vi "Disconnect PV.vi"(8 "error in (no error)":errorcluster, 10 "PV URL":string, 11 "CS++DIMCommandMonitor in":refnum<class "CS++DIMCommandMonitor.lvclass">) -> (0 "error out":errorcluster, 3 "CS++DIMCommandMonitor out":refnum<class "CS++DIMCommandMonitor.lvclass">)   [LabVIEW 2015, in "CS++DIMMonitor.lvlib" / "CS++DIMCommandMonitor.lvclass"]
doc: "Close connection to process variable."
uses:
  CS++DIMCommandMonitor.lvclass
  DIM_Monitor/CS++DIMMonitor.lvclass/CS++DIMMonitor.ctl
  DIM_Monitor/Read DIM IDs.vi
  DIM_Monitor/Read Services.vi
  DIM_Monitor/Write Services.vi
  DIM_Monitor/Write DIM IDs.vi
  DimLVEvent/LVDimInterface/LVDimInterface.lvlib
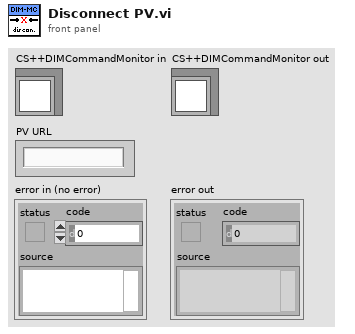
[diagram p1: front panel]
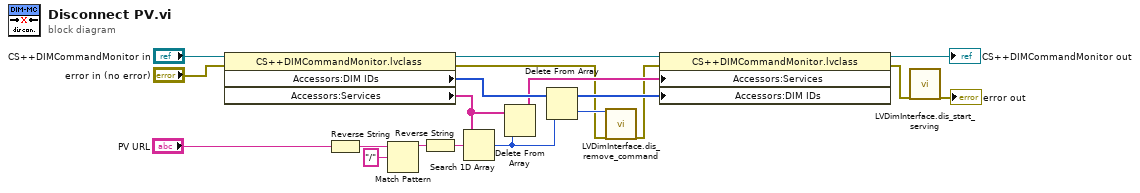
[diagram p0: block diagram]
diagram:
  n1 = property class="CS++DIMCommandMonitor.lvclass"(reference="CS++DIMCommandMonitor in", error in="error in (no error)") -> (reference out=w7:refnum<class "CS++DIMCommandMonitor.lvclass">, error out=w5:errorcluster, "Accessors:DIM IDs"=w11:i32[], "Accessors:Services"=w10:string[])
  n2 = Reverse String(1:"PV URL") -> (0:w18:string)
  n3 = Match Pattern(string=w18, regular expression="/" ("search string/char (-)")) -> (before substring=w17:string)  [unwired: 1 in, 3 out]
  n4 = Reverse String(1:w17) -> (0:w16:string)
  n5 = Search 1D Array(1D array=w10, element=w16) -> (index of element=w15:i32)  [unwired: 1 in]
  n6 = Delete From Array(array=w10, index=w15) -> (array with subset deleted=w9:string[])  [unwired: 1 in, 1 out]
  n7 = Delete From Array(array=w11, index=w15) -> (deleted portion=w6:i32, array with subset deleted=w8:i32[])  [unwired: 1 in]
  n8 = call "LVDimInterface.dis_remove_command.vi"("commandID"=w6, "error in (no error)"=w5) -> ("error out"=w3:errorcluster)  [unwired: 17 in]
  n9 = property class="CS++DIMCommandMonitor.lvclass"(reference=w7, error in=w3, "Accessors:Services"=w9, "Accessors:DIM IDs"=w8) -> (reference out=→"CS++DIMCommandMonitor out":refnum<class "CS++DIMCommandMonitor.lvclass">, error out=w2:errorcluster)
  n10 = call "LVDimInterface.dis_start_serving.vi"("error in (no error)"=w2) -> ("error out"=→"error out":errorcluster)  [unwired: 17 in, 1 out]
